vi "Test Line Intersection with AABB.vi"(11 "Test Case In":refnum<class "Collision Tests.lvclass">) -> (3 "Test Case Out":refnum<class "Collision Tests.lvclass">)   [LabVIEW 2021, in "Collision Tests.lvclass"]
uses:
  Collision Tests.lvclass
  C:/Program Files (x86)/National Instruments/LabVIEW 2026/vi.lib/Astemes/LUnit/Test Case.lvclass
  Re-use Libraries/Vector 2D/Vector 2D.lvclass
  <vilib>/Astemes/LUnit/Test Case.lvclass/Test Case.ctl
  <vilib>/Astemes/LUnit/Test Case.lvclass
  Re-use Libraries/Utility/Typedef/Line.ctl
  Re-use Libraries/Utility/Utility.lvlib
  Re-use Libraries/Collision/Collision.lvlib
  Re-use Libraries/Utility/Typedef/Axis Aligned Bounding Box.ctl
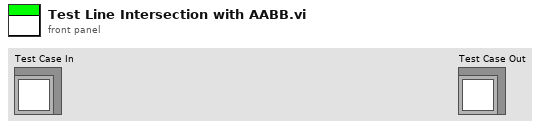
[diagram p1: front panel]
types:
  T1 = typedef "Utility.lvlib/Axis Aligned Bounding Box.ctl" = cluster{"Top Left":refnum<class "Vector 2D.lvclass">, "Bottom Right":refnum<class "Vector 2D.lvclass">}
  T2 = typedef "Utility.lvlib/Line.ctl" = cluster{"Start Point":refnum<class "Vector 2D.lvclass">, "End Point":refnum<class "Vector 2D.lvclass">}
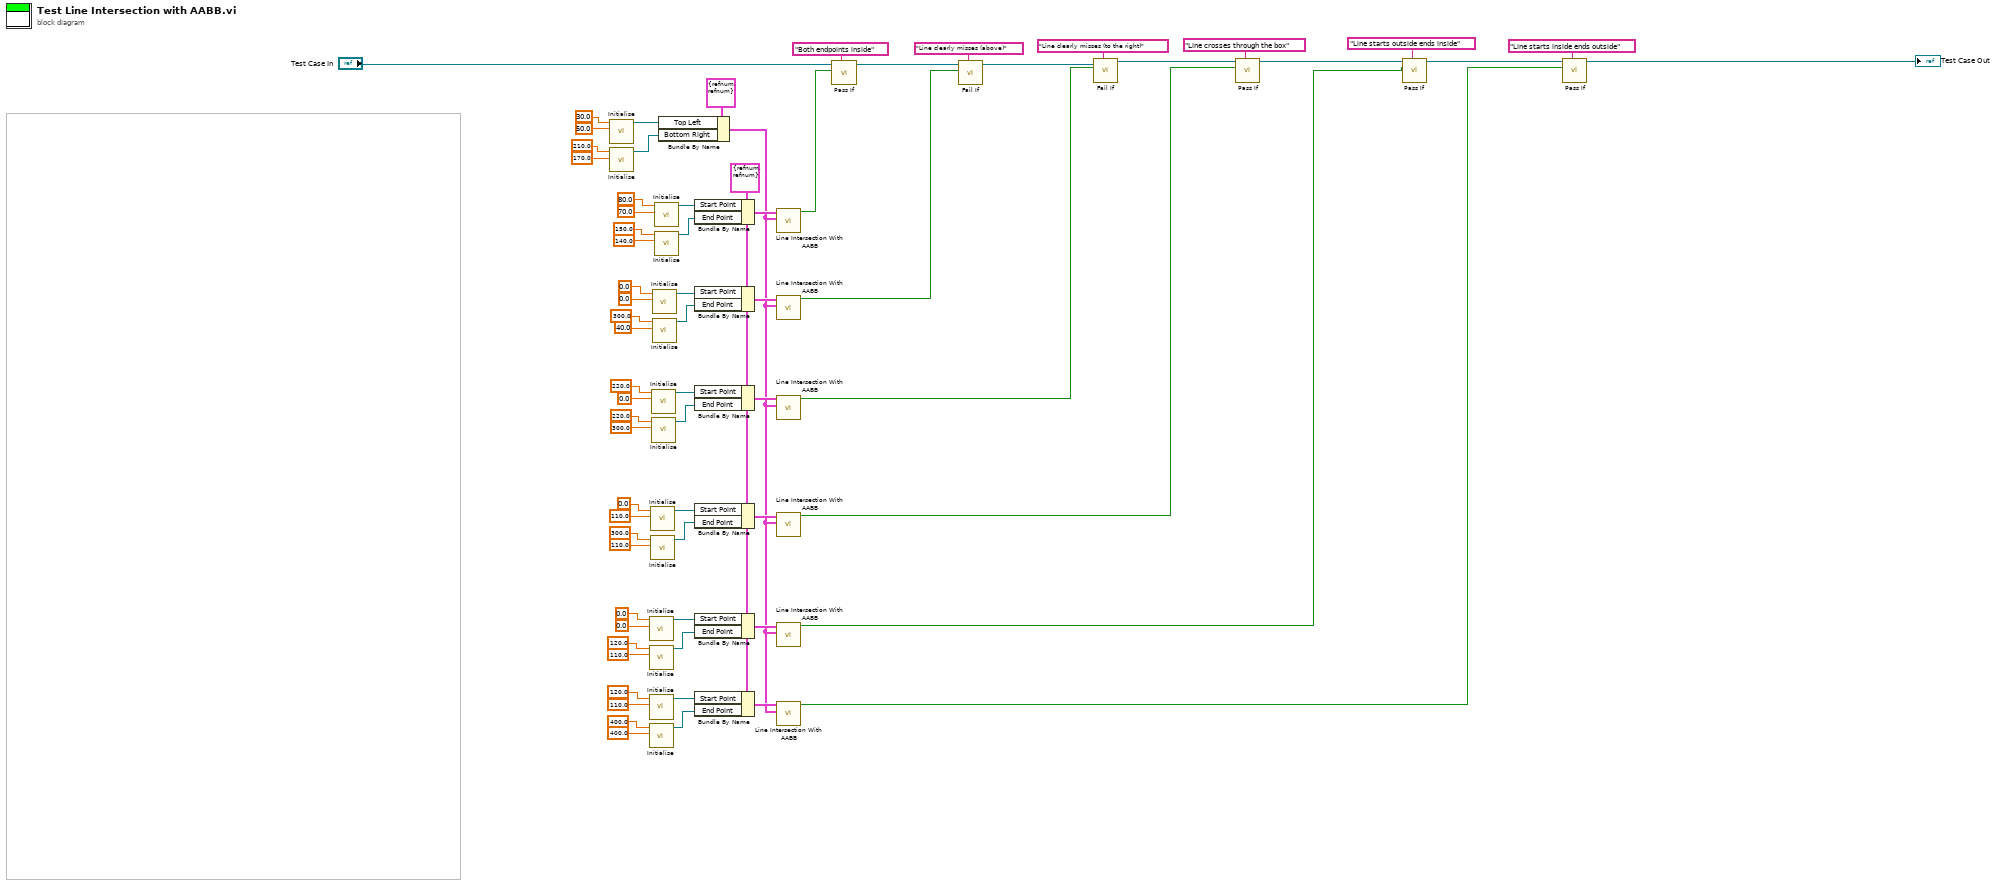
[diagram p0: block diagram]
diagram:
  w4 = T2 {"Start Point"=refnum, "End Point"=refnum} ("Line")
  n1 = call "Initialise.vi"("y"=sgl 50.0 ("x"), "x"=sgl 30.0) -> ("Vector 2D out"=w61:refnum<class "Vector 2D.lvclass">)  [unwired: 9 in]
  n2 = call "Initialise.vi"("y"=sgl 170.0 ("x"), "x"=sgl 210.0) -> ("Vector 2D out"=w60:refnum<class "Vector 2D.lvclass">)  [unwired: 9 in]
  n3 = call "Initialise.vi"("y"=sgl 0.0 ("x"), "x"=sgl 0.0) -> ("Vector 2D out"=w19:refnum<class "Vector 2D.lvclass">)  [unwired: 9 in]
  n4 = call "Initialise.vi"("y"=sgl 110.0 ("x"), "x"=sgl 120.0) -> ("Vector 2D out"=w18:refnum<class "Vector 2D.lvclass">)  [unwired: 9 in]
  n5 = call "Initialise.vi"("y"=sgl 110.0 ("x"), "x"=sgl 120.0) -> ("Vector 2D out"=w7:refnum<class "Vector 2D.lvclass">)  [unwired: 9 in]
  n6 = call "Initialise.vi"("y"=sgl 400.0 ("x"), "x"=sgl 400.0) -> ("Vector 2D out"=w8:refnum<class "Vector 2D.lvclass">)  [unwired: 9 in]
  n7 = call "Initialise.vi"("y"=sgl 110.0 ("x"), "x"=sgl 0.0) -> ("Vector 2D out"=w28:refnum<class "Vector 2D.lvclass">)  [unwired: 9 in]
  n8 = call "Initialise.vi"("y"=sgl 110.0 ("x"), "x"=sgl 300.0) -> ("Vector 2D out"=w29:refnum<class "Vector 2D.lvclass">)  [unwired: 9 in]
  n9 = call "Initialise.vi"("y"=sgl 0.0 ("x"), "x"=sgl 220.0) -> ("Vector 2D out"=w41:refnum<class "Vector 2D.lvclass">)  [unwired: 9 in]
  n10 = call "Initialise.vi"("y"=sgl 300.0 ("x"), "x"=sgl 220.0) -> ("Vector 2D out"=w40:refnum<class "Vector 2D.lvclass">)  [unwired: 9 in]
  n11 = call "Initialise.vi"("y"=sgl 0.0 ("x"), "x"=sgl 0.0) -> ("Vector 2D out"=w49:refnum<class "Vector 2D.lvclass">)  [unwired: 9 in]
  n12 = call "Initialise.vi"("y"=sgl 40.0 ("x"), "x"=sgl 300.0) -> ("Vector 2D out"=w50:refnum<class "Vector 2D.lvclass">)  [unwired: 9 in]
  n13 = call "Initialise.vi"("y"=sgl 70.0 ("x"), "x"=sgl 80.0) -> ("Vector 2D out"=w67:refnum<class "Vector 2D.lvclass">)  [unwired: 9 in]
  n14 = call "Initialise.vi"("y"=sgl 140.0 ("x"), "x"=sgl 150.0) -> ("Vector 2D out"=w66:refnum<class "Vector 2D.lvclass">)  [unwired: 9 in]
  n15 = Bundle By Name(cluster=T1 {"Top Left"=refnum, "Bottom Right"=refnum} ("AABB"), "Top Left"=w61, "Bottom Right"=w60) -> (w3:T1)
  n16 = Bundle By Name(cluster=w4, "Start Point"=w67, "End Point"=w66) -> (w65:T2)
  n17 = Bundle By Name(cluster=w4, "Start Point"=w49, "End Point"=w50) -> (w51:T2)
  n18 = Bundle By Name(cluster=w4, "Start Point"=w41, "End Point"=w40) -> (w39:T2)
  n19 = Bundle By Name(cluster=w4, "Start Point"=w28, "End Point"=w29) -> (w30:T2)
  n20 = Bundle By Name(cluster=w4, "Start Point"=w19, "End Point"=w18) -> (w17:T2)
  n21 = Bundle By Name(cluster=w4, "Start Point"=w7, "End Point"=w8) -> (w9:T2)
  n22 = call "Line Intersection With AABB.vi"("AABB"=w3, "Line"=w65) -> ("Intersects?"=w59:bool)  [unwired: 9 in]
  n23 = call "Line Intersection With AABB.vi"("AABB"=w3, "Line"=w51) -> ("Intersects?"=w45:bool)  [unwired: 9 in]
  n24 = call "Line Intersection With AABB.vi"("AABB"=w3, "Line"=w39) -> ("Intersects?"=w34:bool)  [unwired: 9 in]
  n25 = call "Line Intersection With AABB.vi"("AABB"=w3, "Line"=w30) -> ("Intersects?"=w24:bool)  [unwired: 9 in]
  n26 = call "Line Intersection With AABB.vi"("AABB"=w3, "Line"=w17) -> ("Intersects?"=w14:bool)  [unwired: 9 in]
  n27 = call "Line Intersection With AABB.vi"("AABB"=w3, "Line"=w9) -> ("Intersects?"=w2:bool)  [unwired: 9 in]
  n28 = call <vilib>:"Pass If.vi"("Description"="Both endpoints inside", "Pass?"=w59, "LUnit Test Case In"="Test Case In") -> ("LUnit Test Case Out"=w46:refnum<class "Collision Tests.lvclass">)  [unwired: 7 in, 1 out]
  n29 = call <vilib>:"Fail If.vi"("Description"="Line clearly misses (above)", "Fail?"=w45, "LUnit Test Case In"=w46) -> ("LUnit Test Case Out"=w35:refnum<class "Collision Tests.lvclass">)  [unwired: 7 in, 1 out]
  n30 = call <vilib>:"Fail If.vi"("Description"="Line clearly misses (to the right)", "Fail?"=w34, "LUnit Test Case In"=w35) -> ("LUnit Test Case Out"=w33:refnum<class "Collision Tests.lvclass">)  [unwired: 7 in, 1 out]
  n31 = call <vilib>:"Pass If.vi"("Description"="Line crosses through the box", "Pass?"=w24, "LUnit Test Case In"=w33) -> ("LUnit Test Case Out"=w22:refnum<class "Collision Tests.lvclass">)  [unwired: 7 in, 1 out]
  n32 = call <vilib>:"Pass If.vi"("Description"="Line starts outside ends inside", "Pass?"=w14, "LUnit Test Case In"=w22) -> ("LUnit Test Case Out"=w12:refnum<class "Collision Tests.lvclass">)  [unwired: 7 in, 1 out]
  n33 = call <vilib>:"Pass If.vi"("Description"="Line starts inside ends outside", "Pass?"=w2, "LUnit Test Case In"=w12) -> ("LUnit Test Case Out"=→"Test Case Out":refnum<class "Collision Tests.lvclass">)  [unwired: 7 in, 1 out]
